vi "Tegam4040 - DAC80.vi"(0 "VISA Tegam4040":refnum<visa-resource-name>, 7 "DAC":u16 format="%x", 11 "error in (no error)":errorcluster) -> (4 "VISA Out":refnum<visa-resource-name>, 15 "error out":errorcluster)   [LabVIEW 2010, in "Tegam4040.lvlib"]
doc: "DAC Control:\n\nMust use INIT VI to get DAC in know state of 7FFF. This VI will not read back DAC value as other VI's it will set the Value only."
uses:
  Tegam4040.lvlib
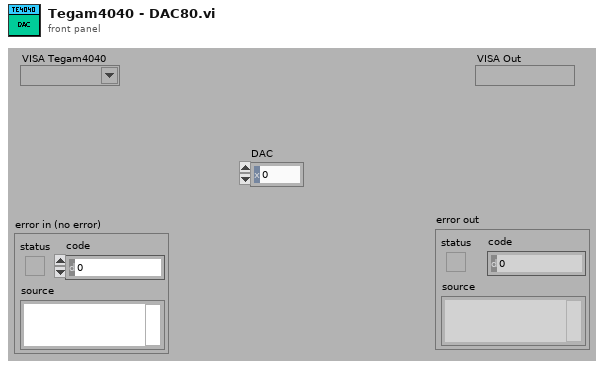
[diagram p1: front panel]
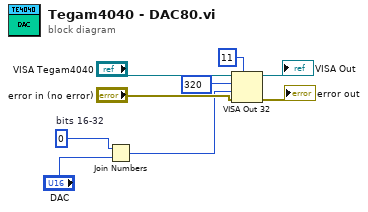
[diagram p0: block diagram]
diagram:
  w2 = u16 0  # bits 16-32
  n1 = Join Numbers(hi=w2, lo="DAC") -> ((hi.lo)=w1:u32)
  n2 = VISA Out 32(7:u16 11 ("address space (A16:  1)"), 8:"error in (no error)", 9:w1, 10:u32 320 ("offset (0)"), 11:"VISA Tegam4040") -> (0:→"error out":errorcluster, 3:→"VISA Out":refnum<visa-resource-name>)
